vi "loop.vi"() -> ()   [LabVIEW 8.6]
panel:
  out "Error Out":errorcluster
  in  "Extension":string
  in  "stop":bool
  out "Output":dbl[](array[numeric])
  out "XY Graph":cluster{timestamp[], dbl[]}[](graph)
  in  "Delimeter":string
  in  "File Name":string
  in  "Label Array":string[](array[string]) caption="Label Array\n(This will be column names of output file)"
  in  "Base Path":path
  in  "Format Array":string[](array[string]) caption="Format Array\n(e.g. %.3f)"
  # "BASIC CONFIGURATIONS"
  # "MEASUREMENT OUTPUTS"
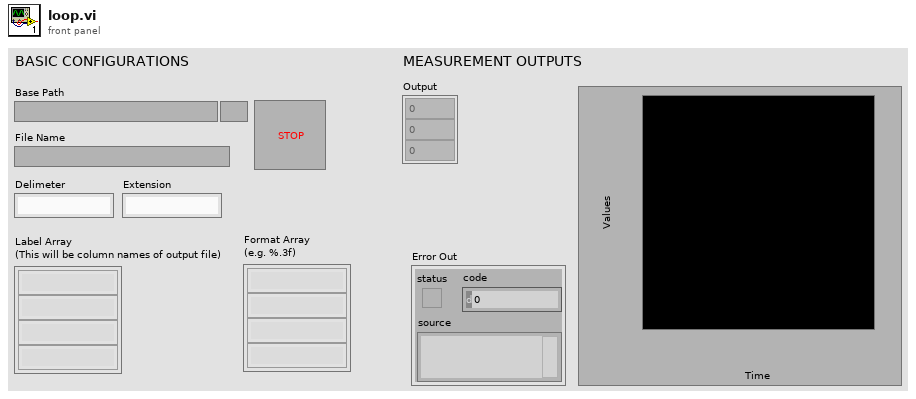
[diagram p1: front panel]
types:
  T1 = enum16{"open", "replace", "create", "open or create", "replace or create", "replace or create with confirmation"}
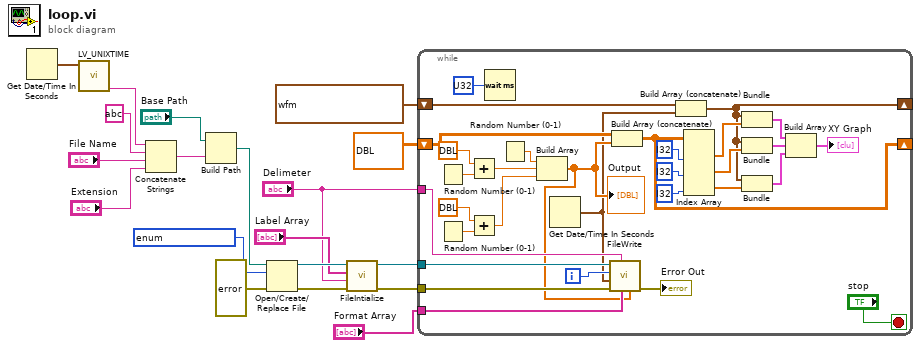
[diagram p0: block diagram]
diagram:
  n1 = Get Date/Time In Seconds() -> (seconds since 1Jan1904=w19:timestamp)
  n2 = call "LV_UNIXTIME.vi"("current time"=w19) -> ("date/time string"=w18:string)  [unwired: 9 in, 1 out]
  n3 = Concatenate Strings(w18, string ? ("string"), "File Name", "Extension") -> (w16:string)
  n4 = Build Path(base path="Base Path", name or relative path=w16) -> (appended path=w15:path)
  n5 = Open/Create/Replace File(file path (use dialog)=w15, error in=errorcluster ?, operation (0:open)=T1 ?) -> (refnum out=w12:refnum<file>, error out=w11:errorcluster)  [unwired: 3 in, 1 out]
  n6 = call "FileIntialize.vi"("Error In"=w11, "Delimeter"="Delimeter", "Labels"="Label Array", "refnum in"=w12) -> ("Error Out"=w9:errorcluster, "File Refnum"=w10:refnum<file>)  [unwired: 6 in]
  n7 = while {
    tunnel: w10 -> [w48]
    tunnel: w9 -> [w47]
    tunnel: "Format Array" -> [w44]
    tunnel: "Delimeter" -> [w45]
    shift-right: [w32] -> _
    shift-left: dbl[][] ? -> [w42]
    shift-right: [w26] -> _
    shift-left: timestamp[] ? -> [w40]
    i -> [w46]
    stop <- "stop" stop-if-true
    n8 = Random Number (0-1)() -> (number: 0 to 1=w38:dbl)
    n9 = Random Number (0-1)() -> (number: 0 to 1=w35:dbl)
    n10 = Add(x=dbl ?, y=w38) -> (x+y=w37:dbl)
    n11 = Add(x=dbl ?, y=w35) -> (x+y=w34:dbl)
    n12 = Wait (ms)(milliseconds to wait=u32 ?) -> ()  [unwired: 1 out]
    n13 = Random Number (0-1)() -> (number: 0 to 1=w49:dbl)
    n14 = Build Array(w49, w37, w34) -> (w43:dbl[])
    "Output" <- w43
    n15 = Get Date/Time In Seconds() -> (seconds since 1Jan1904=w41:timestamp)
    n16 = call "FileWrite.vi"("DataArray"=w43, "FileFormat"=w44, "Delimeter"=w45, "Error In"=w47, "Time Stamp"=w41, "Index"=w46, "refnum in"=w48) -> ("Error Out"=→"Error Out":errorcluster)  [unwired: 3 in, 1 out]
    n17 = Build Array (concatenate)(w42, w43) -> (w32:dbl[][])
    n18 = Build Array (concatenate)(w40, w41) -> (w26:timestamp[])
    n19 = Index Array(array=w32, index (col) #1=i32 ? ("disabled index (col)"), index (col) #2=i32 ? ("disabled index (col)"), index (col) #3=i32 ? ("disabled index (col)")) -> (element #1=w28:dbl[], element #2=w27:dbl[], element #3=w25:dbl[])  [unwired: 3 in]
    n20 = Bundle(w26, w28) -> (w24:cluster{timestamp[], dbl[]})  [unwired: 1 in]
    n21 = Bundle(w26, w27) -> (w23:cluster{timestamp[], dbl[]})  [unwired: 1 in]
    n22 = Bundle(w26, w25) -> (w22:cluster{timestamp[], dbl[]})  [unwired: 1 in]
    n23 = Build Array(w24, w23, w22) -> (→"XY Graph":cluster{timestamp[], dbl[]}[])
  }
